vi "自动数量输出.vi"(11 "选择？":bool) -> ()   [LabVIEW 2010]
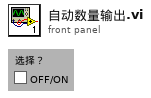
[diagram p1: front panel]
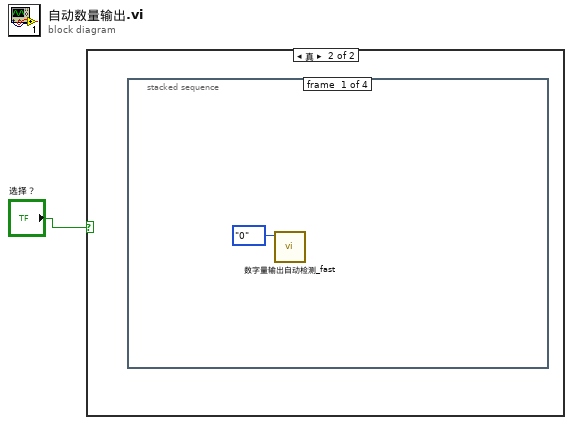
[diagram p0: block diagram]
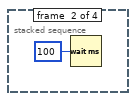
[diagram p3: hidden frame]
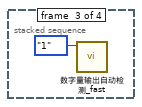
[diagram p4: hidden frame]
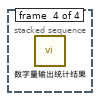
[diagram p5: hidden frame]
diagram:
  n1 = case shown="真" "选择？" {
    frame False {
    }
    frame True {
      n2 = stacked-sequence {
        frame #0 {
          n3 = call "数字量输出自动检测_fast.vi"("测试值"=enum16{"0", "1"}."0") -> ()  [unwired: 11 in]
        }
        frame #1 {
          n4 = Wait (ms)(milliseconds to wait=u32 100 ("等待时间（毫秒）")) -> ()  [unwired: 1 out]
        }
        frame #2 {
          n5 = call "数字量输出自动检测_fast.vi"("测试值"=enum16{"0", "1"}."1") -> ()  [unwired: 11 in]
        }
        frame #3 {
          n6 = call "数字量输出统计结果.vi"() -> ()  [unwired: 12 in]
        }
      }
    }
  }
